vi "current version.vi"() -> ()   [LabVIEW 2014, in "Calculated Tags configuration.lvclass"]
doc: "#CodeRequired\nThis global variable stores the current version of the module and should be updated as serialization formats change."
uses:
  Calculated Tags configuration.lvclass
panel:
  out "current version":string="1.0.0.0"
  # "#MaintenanceRequired update this version whenever the file format (serialization_1_0_0_0.ctl, as an example) changes"
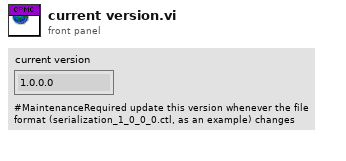
[diagram p1: front panel]
diagram:
